vi "3D Lobatto Quadrature Core.vi"(6 "VI ref":cluster{"f(x)":refnum<vi>, "data":variant}, 7 "formula":string, 9 "tolerance":dbl=1e-10, 10 "Formula/VI ref":bool, 11 "limits":T1={"x limit"={"x lower"=0.0, "x upper"=1.0}, "y limit"={"y lower"=0.0, "y upper"=1.0}, "z limit"={"z lower"=0.0, "z upper"=1.0}}) -> (0 "error out":errorcluster, 3 "result":dbl)   [LabVIEW 2020, in "NI_AALPro.lvlib"]
uses:
  <vilib>/Analysis/NI_AALPro.lvlib
  <vilib>/Analysis/baseanly.llb/A x Vector.vi
  <vilib>/Analysis/baseanly.llb/Real Dot Product.vi
  <vilib>/Analysis/NI_AALBase.lvlib
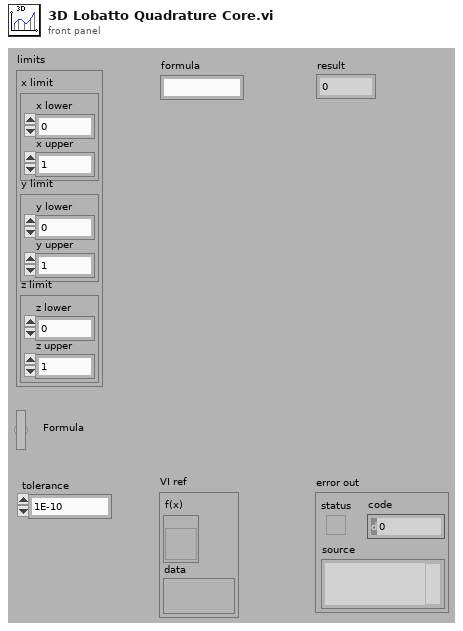
[diagram p1: front panel]
types:
  T1 = cluster{"x limit":cluster{"x lower":dbl, "x upper":dbl}, "y limit":cluster{"y lower":dbl, "y upper":dbl}, "z limit":cluster{"z lower":dbl, "z upper":dbl}}
  T2 = cluster{"x limit":cluster{"x lower":dbl, "x upper":dbl}, "y limit":cluster{"y lower":dbl, "y upper":dbl}, "z limit":cluster{"z lower":dbl, "z upper":dbl}}[]
  T3 = cluster{string[], "Variable Output":string, "formula":string}
  T4 = cluster{"bin x":cluster{"lower limit":dbl, "upper limit":dbl}, "bin y":cluster{"lower limit":dbl, "upper limit":dbl}, "bin z":cluster{"lower limit":dbl, "upper limit":dbl}}[]
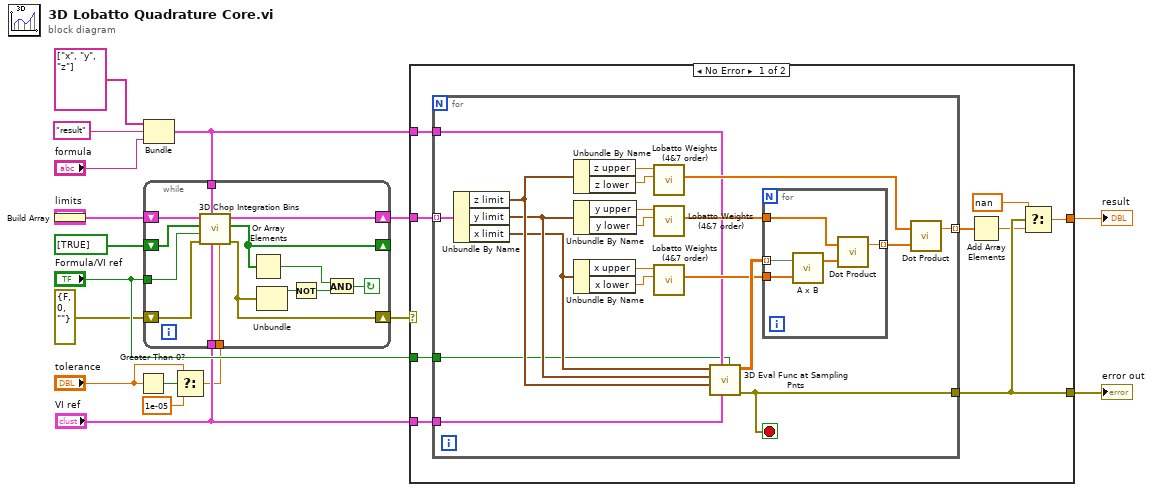
[diagram p0: block diagram]
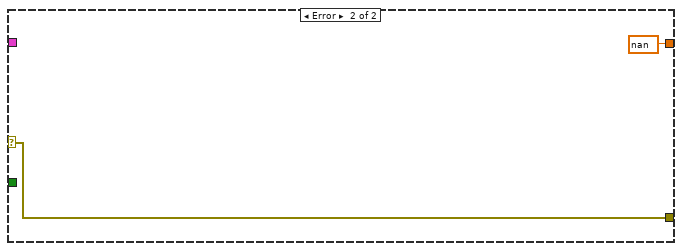
[diagram p2: hidden frame]
diagram:
  n1 = Build Array("limits") -> (w18:T2)
  n2 = Greater Than 0?(x="tolerance") -> (x > 0?=w5:bool)
  n3 = Bundle(string[] ["x", "y", "z"], "Variable Output"="result", "formula"="formula") -> (w7:T3)  [unwired: 1 out]
  n4 = Select(t="tolerance", s=w5, f=1e-05) -> (s? t:f=w2:dbl)
  n5 = while {
    shift-right: [w31] -> w14
    shift-left: w18 -> [w32]
    shift-right: [w29] -> _
    shift-left: bool[] [TRUE] ("appended array") -> [w30]
    tunnel: w7 -> [w28]
    tunnel: "Formula/VI ref" -> [w25]
    tunnel: w2 -> [w27]
    tunnel: "VI ref" -> [w26]
    shift-right: [w23] -> w1
    shift-left: errorcluster {"status"=FALSE, "code"=0, "source"=""} ("error out") -> [w24]
    stop <- w19 continue-if-true
    n6 = call <vilib>:"3D Chop Integration Bins.vi"("tolerance"=w27, "VI ref"=w26, "Formula"=w28, "error in (no error)"=w24, "Formula/VI ref"=w25, "Chop In"=w30, "Bins In"=w32) -> ("error out"=w23:errorcluster, "Chop Out"=w29:bool[], "Bins Out"=w31:T4)  [unwired: 2 out]
    n7 = Or Array Elements(Boolean array=w29) -> (logical OR=w20:bool)
    n8 = Unbundle(w23) -> ("status"=w22:bool)  [unwired: 2 out]
    n9 = Not(x=w22) -> (.not. x?=w21:bool)
    n10 = And(x=w20, y=w21) -> (x .and. y?=w19:bool)
  }
  n11 = case shown="No Error" w1 {
    selector: w1 -> [_ w68]
    tunnel: [w33 nan ("X * Y")] -> w17
    tunnel: w14 -> [w41 _]
    tunnel: [w36 w68] -> w13
    tunnel: "Formula/VI ref" -> [w39 _]
    tunnel: "VI ref" -> [w38 _]
    tunnel: w7 -> [w37 _]
    frame No Error {
      n12 = for {
        tunnel: w41 -> [w49] mode=indexing
        tunnel: [w52] -> w40 mode=indexing
        tunnel: w37 -> [w45]
        tunnel: w39 -> [w44]
        tunnel: w38 -> [w43]
        tunnel: [w42] -> w36
        stop <- w42 stop-if-true
        n13 = Unbundle By Name(w49) -> ("z limit"=w48:cluster{"z lower":dbl, "z upper":dbl}, "y limit"=w47:cluster{"y lower":dbl, "y upper":dbl}, "x limit"=w46:cluster{"x lower":dbl, "x upper":dbl})
        n14 = Unbundle By Name(w48) -> ("z upper"=w51:dbl, "z lower"=w50:dbl)
        n15 = Unbundle By Name(w47) -> ("y upper"=w60:dbl, "y lower"=w59:dbl)
        n16 = Unbundle By Name(w46) -> ("x upper"=w57:dbl, "x lower"=w56:dbl)
        n17 = call <vilib>:"Lobatto Weights (4&7 order).vi"("lower limit"=w50, "upper limit"=w51) -> ("Weights (7-Order)"=w53:dbl[])  [unwired: 9 out]
        n18 = call <vilib>:"Lobatto Weights (4&7 order).vi"("lower limit"=w59, "upper limit"=w60) -> ("Weights (7-Order)"=w58:dbl[])  [unwired: 9 out]
        n19 = call <vilib>:"Lobatto Weights (4&7 order).vi"("lower limit"=w56, "upper limit"=w57) -> ("Weights (7-Order)"=w55:dbl[])  [unwired: 9 out]
        n20 = call <vilib>:"3D Eval Func at Sampling Pnts.vi"("Formula/VI ref"=w44, "VI ref"=w43, "Formula"=w45, "z limit"=w48, "y limit"=w47, "x limit"=w46) -> ("error out"=w42:errorcluster, "Function Evaluations (7 pts)"=w61:dbl[][][])  [unwired: 1 in, 3 out]
        n21 = for {
          tunnel: w61 -> [w64] mode=indexing
          tunnel: w58 -> [w66]
          tunnel: [w65] -> w54 mode=indexing
          tunnel: w55 -> [w63]
          n22 = call-poly <vilib>:"A x B.vi"("Vector"=w63, "A"=w64) -> ("A x Vector"=w62:dbl[])  [unwired: 1 out]
          n23 = call-poly <vilib>:"Dot Product.vi"("Y Vector"=w62, "X Vector"=w66) -> ("X * Y"=w65:dbl)  [unwired: 1 out]
        }
        n24 = call-poly <vilib>:"Dot Product.vi"("Y Vector"=w54, "X Vector"=w53) -> ("X * Y"=w52:dbl)  [unwired: 1 out]
      }
      n25 = Add Array Elements(numeric array=w40) -> (sum=w34:dbl)
      n26 = Select(t=nan, s=w36, f=w34) -> (s? t:f=w33:dbl)
    }
    frame Error {
    }
  }
  "result" <- w17
  "error out" <- w13
